vi "Tag.index_lua.vi"(5 "LuaVIEW reference":T1) -> (15 "error out":errorcluster)   [LabVIEW 2012]
doc: "Set the read_index relative to the write position. This changes the read position in the tag buffer that will be used during the next <code>read</code>. When delta is zero, the read_index is set to the next point to be written. When the delta is negative and equals -N, the read_index will point to the Nth most recently written point. When the delta is positive and equals N, N upcoming points will be skipped. Note that the number of available earlier points equals the minimum of either the tag's buffer capacity or the number of written points. Therefore do not move the read_index backward too far or else the subsequent <code>read</code> will fail.\nParameters:\nobj:tag\nI32:delta, number of point positions by which to change the read_index.\nErrors:\nDead or invalid tag object.\nData logger not initialized."
uses:
  luaview/typedefs/t_LuaVIEW Reference.ctl
  typedefs/t_DataLog Tag Buffers Methods.ctl
  luaview/subvis/private/LuaVIEW Pull (object).vi
  luaview/subvis/private/LuaVIEW Pull (I32).vi
  luaview/subvis/private/LuaVIEW Push (I32).vi
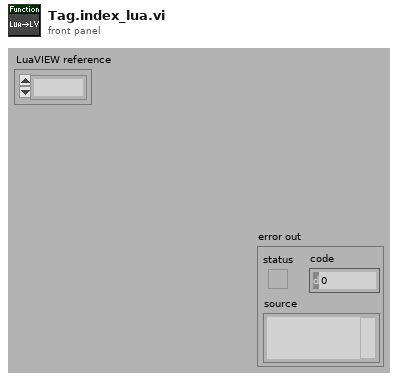
[diagram p1: front panel]
types:
  T1 = typedef "t_LuaVIEW Reference.ctl" = refnum<k1>
  T2 = typedef "t_DataLog Tag Buffers Methods.ctl" = enum16{"initialize", "inert", "write", "read", "read oldest", "read last", "cleanup"}
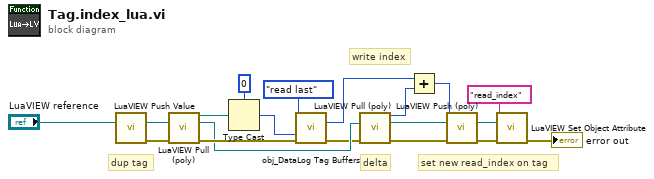
[diagram p0: block diagram]
diagram:
  # "write index"
  # "delta"
  # "set new read_index on tag"
  # "dup tag"
  n1 = call "LuaVIEW Push Value.vi"("LuaVIEW reference in"="LuaVIEW reference") -> ("LuaVIEW reference out"=w19:T1, "error out"=w18:errorcluster)  [unwired: 13 in]
  n2 = call-poly "LuaVIEW Pull (poly).vi"("LuaVIEW reference in"=w19, "error in (no error)"=w18) -> ("object refnum"=w11:refnum<vi>, "LuaVIEW reference out"=w3:T1, "error out"=w6:errorcluster)  [unwired: 10 in, 1 out]
  n3 = Type Cast(type=0 ("read index in"), x=w11) -> (*(type *) &x=w2:i32)
  n4 = call "obj_DataLog Tag Buffers.vi"("method"=t_DataLog_Tag_Buffers_Methods."read last", "tag index"=w2, "error in (no error)"=w6) -> ("read index out"=w4:i32, "error out"=w1:errorcluster)  [unwired: 8 in, 3 out]
  n5 = call-poly "LuaVIEW Pull (poly).vi"("LuaVIEW reference in"=w3, "error in (no error)"=w1) -> ("I32"=w9:i32, "LuaVIEW reference out"=w8:T1, "error out"=w7:errorcluster)  [unwired: 11 in]
  n6 = Add(x=w4, y=w9) -> (x+y=w14:i32)
  n7 = call-poly "LuaVIEW Push (poly).vi"("I32"=w14, "LuaVIEW reference in"=w8, "error in (no error)"=w7) -> ("LuaVIEW reference out"=w16:T1, "error out"=w17:errorcluster)  [unwired: 11 in]
  n8 = call "LuaVIEW Set Object Attribute.vi"("key"="read_index", "LuaVIEW reference in"=w16, "error in (no error)"=w17) -> ("error out"=→"error out":errorcluster)  [unwired: 11 in, 1 out]
